vi "LVClass_WavefrontCorrectorSet Set WavefrontCorrectorParameter.vi"(0 "WavefrontCorrectorSet in":refnum<class "WavefrontCorrectorSet.lvclass">, 5 "CameraParametersSettable":T1[](array[typedef]), 11 "error in (no error)":errorcluster) -> (4 "WavefrontCorrectorSet out":refnum<class "WavefrontCorrectorSet.lvclass">, 15 "error out":errorcluster)   [LabVIEW 2020, in "WavefrontCorrectorSet.lvclass"]
doc: "WavefrontCorrector parameter default value getter for parameter of type\nboolean.\n\n--------------------------------------------------------------------------------\n\n<B>wavefrontcorrector_setIn </B> : WavefrontCorrectorSet object.\n<B>wavefrontcorrector_setOut </B> : WavefrontCorrectorSet object.\n<B>parameter_name </B> : Parameter name.\n<B>default_value </B> : Parameter default value.\n<B>ErrorIn </B> : Error\n<B>ErrorOut </B> : Error\n\n--------------------------------------------------------------------------------"
uses:
  WavefrontCorrectorSet.lvclass
  CameraParametersSetup.ctl
  CameraParameters_Type.ctl
  WavefrontCorrectorSet.lvclass/WavefrontCorrectorSet.ctl
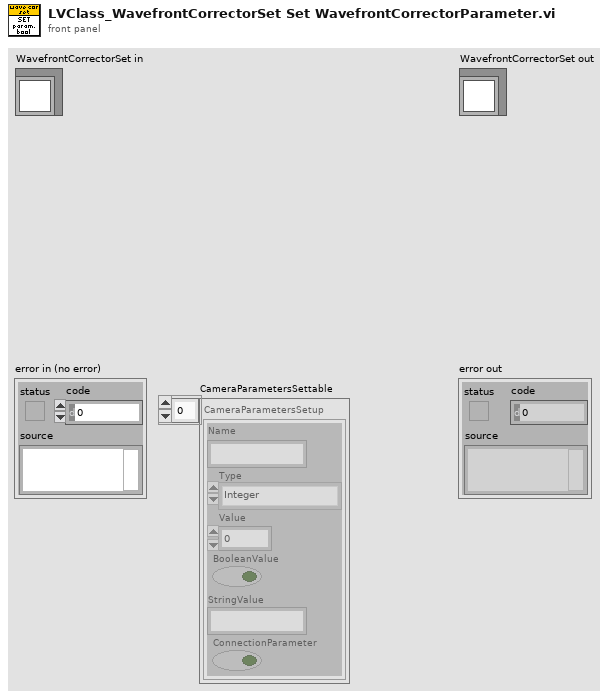
[diagram p1: front panel]
types:
  T1 = typedef "CameraParametersSetup.ctl" = cluster{"Name":string, "Type":T2, "Value":dbl, "BooleanValue":bool, "StringValue":string, "ConnectionParameter":bool}
  T2 = typedef "CameraParameters_Type.ctl" = enum16{"Integer", "Real", "String", "Boolean"}
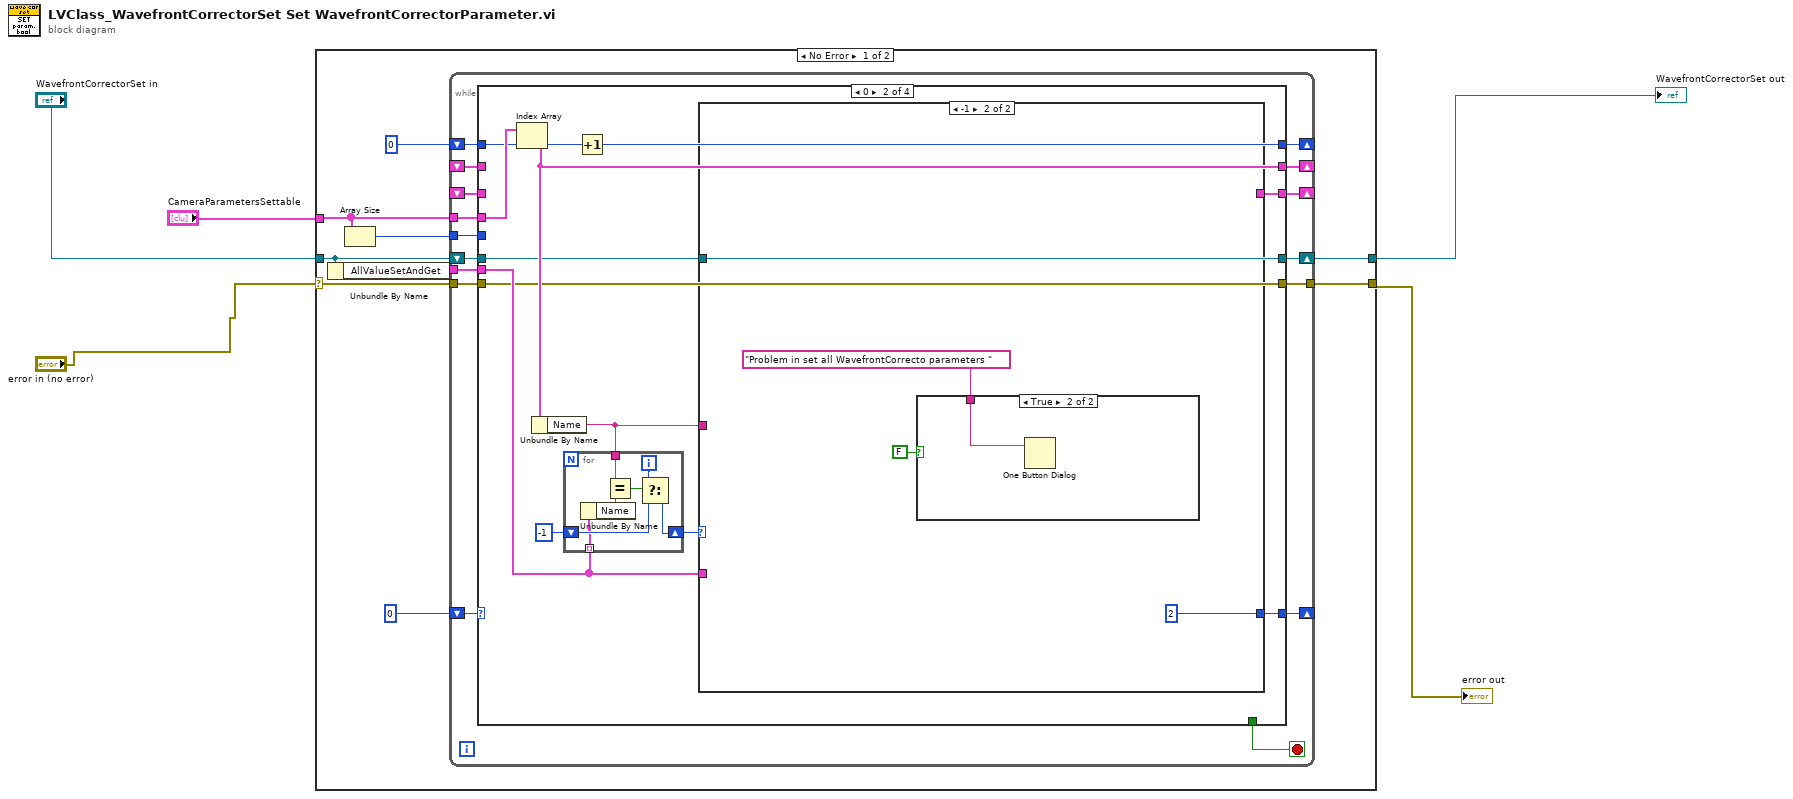
[diagram p0: block diagram]
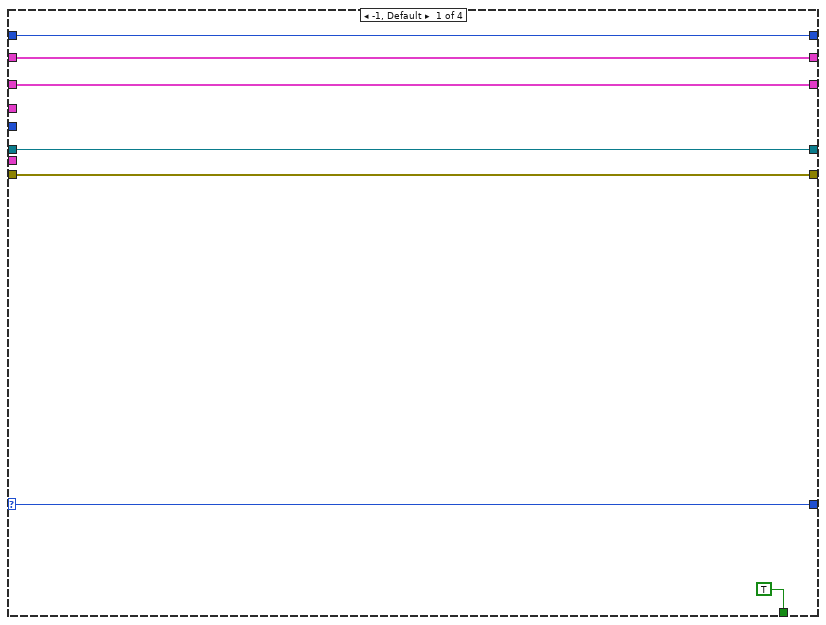
[diagram p2: hidden frame]
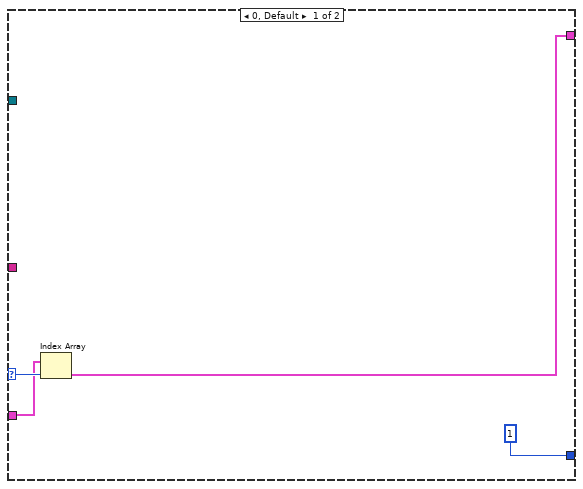
[diagram p3: hidden frame]
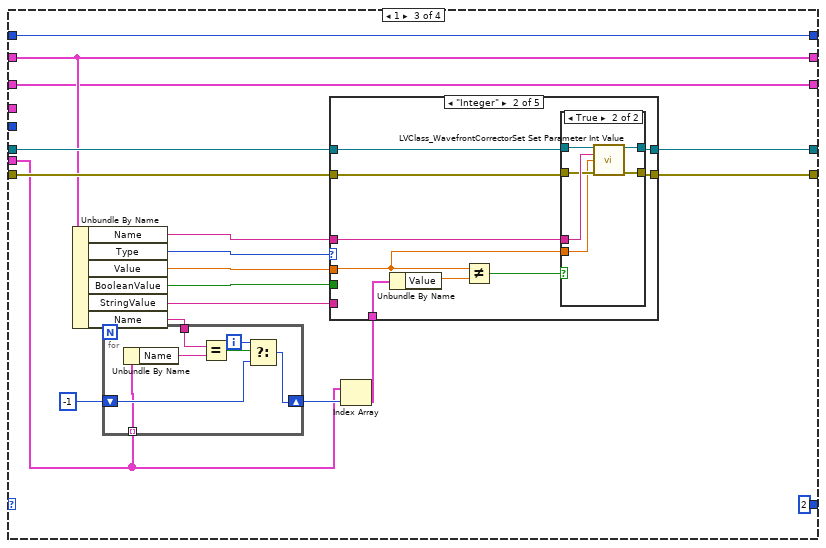
[diagram p5: hidden frame]
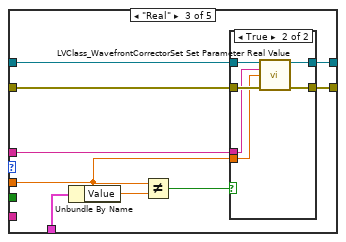
[diagram p8: hidden frame]
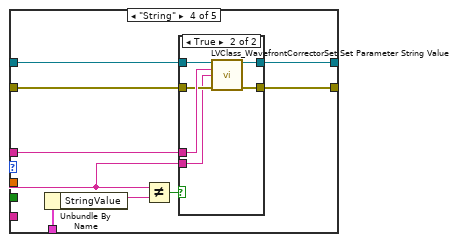
[diagram p10: hidden frame]
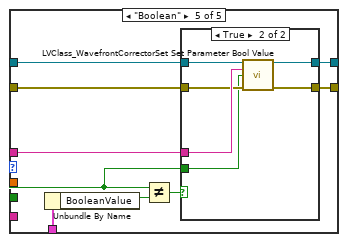
[diagram p12: hidden frame]
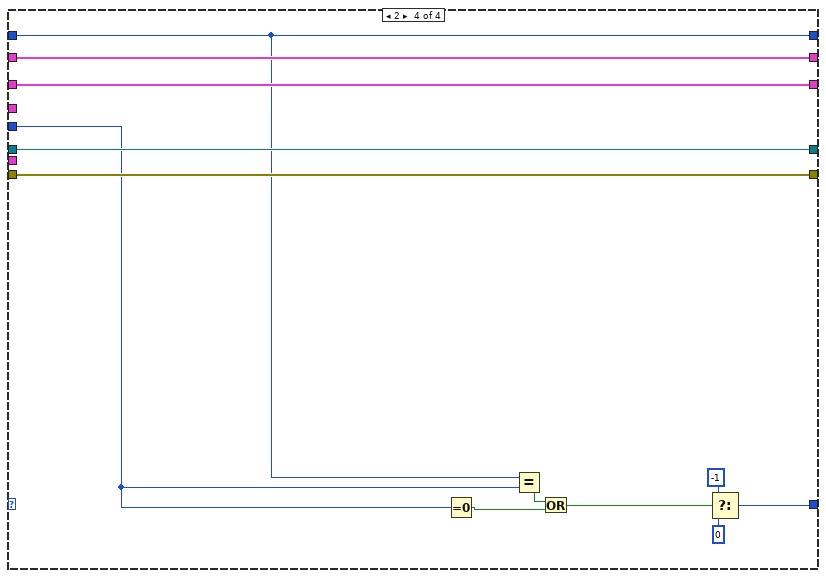
[diagram p14: hidden frame]
diagram:
  n1 = case shown="No Error" "error in (no error)" {
    selector: "error in (no error)" -> [w6 w173]
    tunnel: [w12 w173] -> w1
    tunnel: [w13 w172] -> w2
    tunnel: "WavefrontCorrectorSet in" -> [w7 w172]
    tunnel: "CameraParametersSettable" -> [w10 _]
    frame No Error {
      n2 = Unbundle By Name(w7) -> ("AllValueSetAndGet"=w8:T1[])
      n3 = Array Size(array=w10) -> (size(s)=w9:i32)
      n4 = while {
        tunnel: w6 -> [w26]
        shift-right: [w29] -> _
        shift-left: 0 -> [w30]
        tunnel: w8 -> [w24]
        tunnel: [w25] -> w12
        tunnel: w10 -> [w23]
        shift-right: [w27] -> w13
        shift-left: w7 -> [w28]
        shift-right: [w18] -> _
        shift-left: 0 -> [w21]
        shift-right: [w20] -> _
        shift-left: _ -> [w19]
        tunnel: w9 -> [w17]
        shift-right: [w16] -> _
        shift-left: _ -> [w15]
        stop <- w22 stop-if-true
        n5 = case shown="0" w30 {
          selector: w30 -> [w31 _ _ _]
          tunnel: [w31 w42 2 w166] -> w29
          tunnel: w28 -> [w37 w41 w81 w169]
          tunnel: [w37 w41 w80 w169] -> w27
          tunnel: w26 -> [w36 w44 w79 w168]
          tunnel: [w36 w44 w78 w168] -> w25
          tunnel: w24 -> [_ w49 w65 _]
          tunnel: w23 -> [_ w46 _ _]
          tunnel: [TRUE _ _ _] -> w22
          tunnel: w21 -> [w32 w43 w68 w167]
          tunnel: [w34 w45 w77 w171] -> w20
          tunnel: w19 -> [w34 _ w77 w171]
          tunnel: [w32 w39 w68 w167] -> w18
          tunnel: w17 -> [_ _ _ w163]
          tunnel: [w33 w38 w66 w170] -> w16
          tunnel: w15 -> [w33 _ w66 w170]
          frame -1, Default {
          }
          frame 0 {
            n6 = Index Array(array=w46, index=w43) -> (element=w45:T1)
            n7 = Unbundle By Name(w45) -> ("Name"=w40:string)
            n8 = for {
              tunnel: w40 -> [w63]
              shift-right: [w60] -> w47
              shift-left: -1 -> [w59]
              tunnel: w49 -> [w58] mode=indexing
              i -> [w61]
              n9 = Unbundle By Name(w58) -> ("Name"=w64:string)
              n10 = Equal?(x=w63, y=w64) -> (x = y?=w62:bool)
              n11 = Select(t=w61, s=w62, f=w59) -> (s? t:f=w60:i32)
            }
            n12 = Increment(x=w43) -> (x+1=w39:i32)
            n13 = case shown="-1" w47 {
              selector: w47 -> [w53 _]
              tunnel: w49 -> [w52 _]
              tunnel: [1 2] -> w42
              tunnel: w41 -> [_ _]
              tunnel: w40 -> [_ _]
              tunnel: [w51 _] -> w38
              frame 0, Default {
                n14 = Index Array(array=w52, index=w53) -> (element=w51:T1)
              }
              frame -1 {
                n15 = case shown="True" FALSE {
                  tunnel: "Problem in set all WavefrontCorrecto parameters " ("message") -> [_ w57]
                  frame False {
                  }
                  frame True {
                    n16 = One Button Dialog(message=w57) -> ()  [unwired: 1 in, 1 out]
                  }
                }
              }
            }
          }
          frame 1 {
            n17 = Unbundle By Name(w77) -> ("Name"=w71:string, "Type"=w76:T2, "Value"=w72:dbl, "BooleanValue"=w74:bool, "StringValue"=w73:string, "Name"=w70:string)
            n18 = for {
              tunnel: w70 -> [w158]
              shift-right: [w155] -> w69
              shift-left: -1 -> [w154]
              tunnel: w65 -> [w153] mode=indexing
              i -> [w156]
              n19 = Unbundle By Name(w153) -> ("Name"=w159:string)
              n20 = Equal?(x=w158, y=w159) -> (x = y?=w157:bool)
              n21 = Select(t=w156, s=w157, f=w154) -> (s? t:f=w155:i32)
            }
            n22 = Index Array(array=w65, index=w69) -> (element=w67:T1)
            n23 = case shown="\"Integer\"" w76 {
              tunnel: w71 -> [_ w86 w103 w125 w142]
              tunnel: w81 -> [w84 w92 w109 w126 w143]
              tunnel: [w84 w90 w107 w123 w140] -> w80
              tunnel: [w83 w89 w106 w122 w139] -> w78
              tunnel: w79 -> [w83 w91 w108 w124 w141]
              tunnel: w67 -> [_ w93 w110 w127 w144]
              tunnel: w72 -> [_ w88 w104 _ _]
              tunnel: w74 -> [_ _ _ _ w136]
              tunnel: w73 -> [_ _ _ w119 _]
              frame Default {
              }
              frame "Integer" {
                n24 = Unbundle By Name(w93) -> ("Value"=w87:dbl)
                n25 = Not Equal?(x=w88, y=w87) -> (x != y?=w85:bool)
                n26 = case shown="True" w85 {
                  tunnel: w92 -> [w95 w101]
                  tunnel: w86 -> [_ w100]
                  tunnel: w91 -> [w94 w99]
                  tunnel: [w95 w98] -> w90
                  tunnel: [w94 w97] -> w89
                  tunnel: w88 -> [_ w96]
                  frame False {
                  }
                  frame True {
                    n27 = call "LVClass_WavefrontCorrectorSet Set Parameter Int Value.vi"("WavefrontCorrectorSet in"=w101, "parameter_name"=w100, "Value"=w96, "error in (no error)"=w99) -> ("WavefrontCorrectorSet out"=w98:refnum<class "WavefrontCorrectorSet.lvclass">, "error out"=w97:errorcluster)  [unwired: 10 in]
                  }
                }
              }
              frame "Real" {
                n28 = Unbundle By Name(w110) -> ("Value"=w105:dbl)
                n29 = Not Equal?(x=w104, y=w105) -> (x != y?=w102:bool)
                n30 = case shown="True" w102 {
                  tunnel: w109 -> [w112 w118]
                  tunnel: w103 -> [_ w114]
                  tunnel: w108 -> [w111 w115]
                  tunnel: [w112 w117] -> w107
                  tunnel: [w111 w116] -> w106
                  tunnel: w104 -> [_ w113]
                  frame False {
                  }
                  frame True {
                    n31 = call "LVClass_WavefrontCorrectorSet Set Parameter Real Value.vi"("WavefrontCorrectorSet in"=w118, "parameter_name"=w114, "Value"=w113, "error in (no error)"=w115) -> ("WavefrontCorrectorSet out"=w117:refnum<class "WavefrontCorrectorSet.lvclass">, "error out"=w116:errorcluster)  [unwired: 10 in]
                  }
                }
              }
              frame "String" {
                n32 = Unbundle By Name(w127) -> ("StringValue"=w120:string)
                n33 = Not Equal?(x=w119, y=w120) -> (x != y?=w121:bool)
                n34 = case shown="True" w121 {
                  tunnel: w126 -> [w129 w135]
                  tunnel: w125 -> [_ w132]
                  tunnel: w124 -> [w128 w131]
                  tunnel: [w129 w134] -> w123
                  tunnel: [w128 w133] -> w122
                  tunnel: w119 -> [_ w130]
                  frame False {
                  }
                  frame True {
                    n35 = call "LVClass_WavefrontCorrectorSet Set Parameter String Value.vi"("WavefrontCorrectorSet in"=w135, "parameter name"=w132, "Value"=w130, "error in (no error)"=w131) -> ("WavefrontCorrectorSet out"=w134:refnum<class "WavefrontCorrectorSet.lvclass">, "error out"=w133:errorcluster)  [unwired: 10 in]
                  }
                }
              }
              frame "Boolean" {
                n36 = Unbundle By Name(w144) -> ("BooleanValue"=w137:bool)
                n37 = Not Equal?(x=w136, y=w137) -> (x != y?=w138:bool)
                n38 = case shown="True" w138 {
                  tunnel: w143 -> [w146 w152]
                  tunnel: w142 -> [_ w150]
                  tunnel: w141 -> [w145 w149]
                  tunnel: [w146 w151] -> w140
                  tunnel: [w145 w148] -> w139
                  tunnel: w136 -> [_ w147]
                  frame False {
                  }
                  frame True {
                    n39 = call "LVClass_WavefrontCorrectorSet Set Parameter Bool Value.vi"("WavefrontCorrectorSet in"=w152, "parameter_name"=w150, "Value"=w147, "error in (no error)"=w149) -> ("WavefrontCorrectorSet out"=w151:refnum<class "WavefrontCorrectorSet.lvclass">, "error out"=w148:errorcluster)  [unwired: 10 in]
                  }
                }
              }
            }
          }
          frame 2 {
            n40 = Equal To 0?(x=w163) -> (x = 0?=w162:bool)
            n41 = Equal?(x=w167, y=w163) -> (x = y?=w161:bool)
            n42 = Or(x=w161, y=w162) -> (x .or. y?=w160:bool)
            n43 = Select(t=-1, s=w160, f=0) -> (s? t:f=w166:i32)
          }
        }
      }
    }
    frame Error {
    }
  }
  "error out" <- w1
  "WavefrontCorrectorSet out" <- w2
